vi "total.vi"(8 "count":i32, 10 "discount":dbl format="%#_13g", 11 "size":dbl format="%#_13g") -> (2 "price":i32)   [LabVIEW 2023]
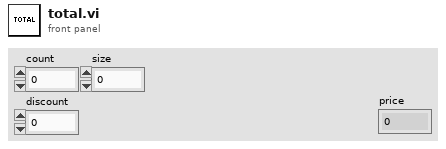
[diagram p1: front panel]
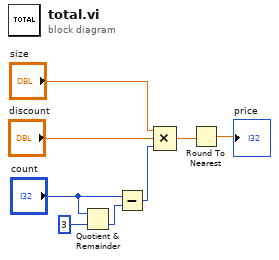
[diagram p0: block diagram]
diagram:
  n1 = Quotient & Remainder(x="count", y=3) -> (floor(x/y)=w7:i32)  [unwired: 1 out]
  n2 = Subtract(x="count", y=w7) -> (x-y=w5:i32)
  n3 = Compound Arithmetic op=MULTIPLY("size", "discount", w5) -> (w6:dbl)
  n4 = Round To Nearest(number=w6) -> (nearest integer value=→"price":dbl)
